vi "Timing.vi"(8 "error in":errorcluster, 9 "Stabilization Interval (s)":dbl, 10 "Time Left":refnum<notifier>, 11 "Message Queues out":T2) -> (0 "error out":errorcluster)   [LabVIEW 2014, in "Timing and Stabilization.lvlib"]
uses:
  Timing and Stabilization.lvlib
  MeasurementControl Message Queue Folder/All Message Queues.ctl
  MeasurementControl Message Queue Folder/Message Cluster.ctl
  Time Left.ctl
  MeasurementControl Message Queue Folder/Enqueue Message (Single).vi
  MeasurementControl Message Queue Folder/MeasurementControl Message Queue.lvlib
panel:
  out "Cluster":T1
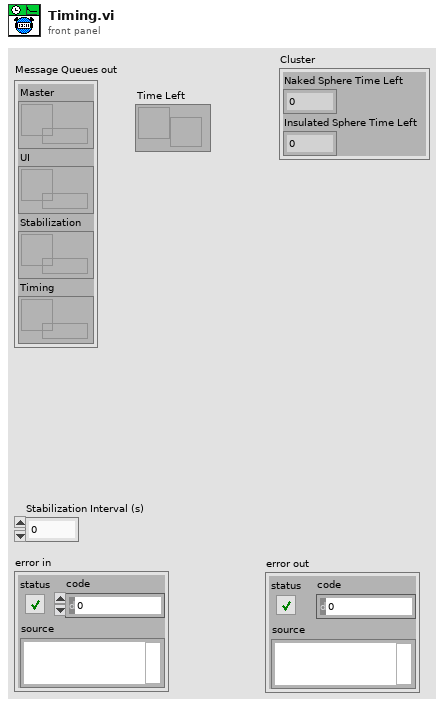
[diagram p1: front panel]
types:
  T1 = typedef "Time Left.ctl" = cluster{"Naked Sphere Time Left":dbl, "Insulated Sphere Time Left":dbl}
  T2 = typedef "MeasurementControl Message Queue.lvlib/All Message Queues.ctl" = cluster{"Master":refnum<queue>, "UI":refnum<queue>, "Stabilization":refnum<queue>, "Timing":refnum<queue>}
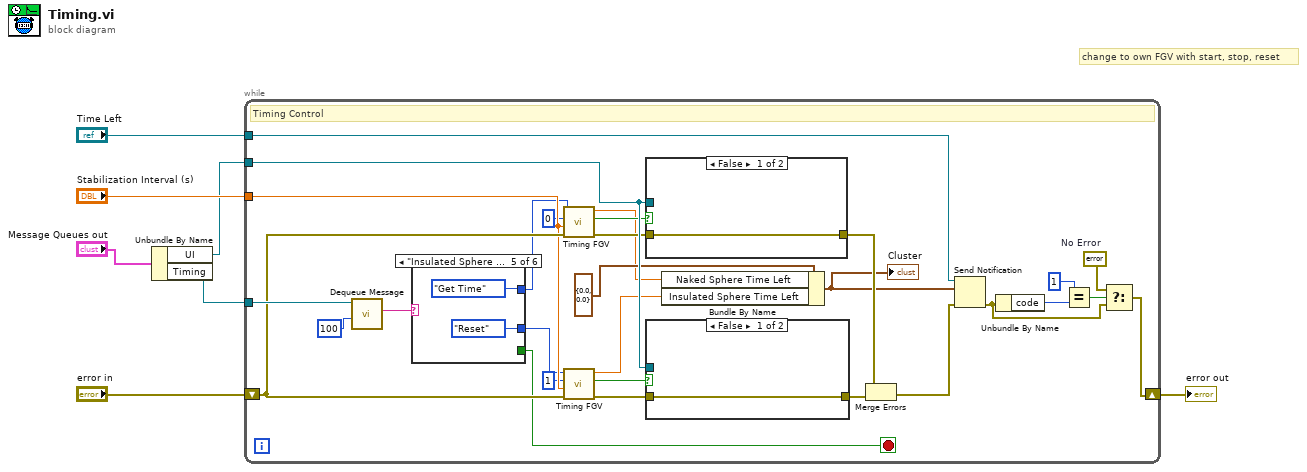
[diagram p0: block diagram]
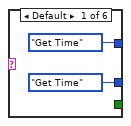
[diagram p2: hidden frame]
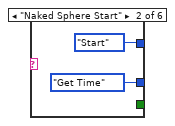
[diagram p3: hidden frame]
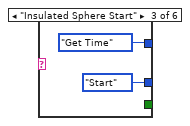
[diagram p4: hidden frame]
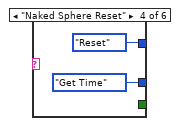
[diagram p5: hidden frame]
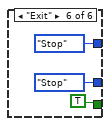
[diagram p6: hidden frame]
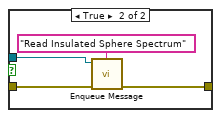
[diagram p7: hidden frame]
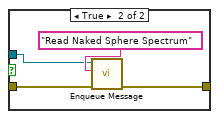
[diagram p8: hidden frame]
diagram:
  # "change to own FGV with start, stop, reset"
  n1 = Unbundle By Name("Message Queues out") -> ("UI"=w3:refnum<queue>, "Timing"=w2:refnum<queue>)
  n2 = while {
    shift-right: [w8] -> w5
    shift-left: "error in" -> [w31]
    tunnel: w2 -> [w36]
    tunnel: "Stabilization Interval (s)" -> [w28]
    tunnel: w3 -> [w33]
    tunnel: "Time Left" -> [w15]
    stop <- w20 stop-if-true
    w10 = errorcluster {"status"=FALSE, "code"=0, "source"=""}  # No Error
    # "Timing Control"
    n3 = call "Dequeue Message.vi"("timeout in ms (-1)"=100, "Message Queue"=w36) -> ("Message"=w23:string)  [unwired: 6 in, 3 out]
    n4 = case shown="\"Insulated Sphere Reset\"" w23 {
      tunnel: [enum16{"Start", "Stop", "Reset", "Get Time"}."Get Time" ("Method (Get Time)") enum16{"Start", "Stop", "Reset", "Get Time"}."Start" ("Method (Get Time)") enum16{"Start", "Stop", "Reset", "Get Time"}."Get Time" ("Method (Get Time)") enum16{"Start", "Stop", "Reset", "Get Time"}."Reset" ("Method (Get Time)") enum16{"Start", "Stop", "Reset", "Get Time"}."Get Time" ("Method (Get Time)") enum16{"Start", "Stop", "Reset", "Get Time"}."Stop" ("Method (Get Time)")] -> w22
      tunnel: [enum16{"Start", "Stop", "Reset", "Get Time"}."Get Time" ("Method (Get Time)") enum16{"Start", "Stop", "Reset", "Get Time"}."Get Time" ("Method (Get Time)") enum16{"Start", "Stop", "Reset", "Get Time"}."Start" ("Method (Get Time)") enum16{"Start", "Stop", "Reset", "Get Time"}."Get Time" ("Method (Get Time)") enum16{"Start", "Stop", "Reset", "Get Time"}."Reset" ("Method (Get Time)") enum16{"Start", "Stop", "Reset", "Get Time"}."Stop" ("Method (Get Time)")] -> w21
      tunnel: [_ _ _ _ _ TRUE] -> w20
      frame Default {
      }
      frame "Naked Sphere Start" {
      }
      frame "Insulated Sphere Start" {
      }
      frame "Naked Sphere Reset" {
      }
      frame "Insulated Sphere Reset" {
      }
      frame "Exit" {
      }
    }
    n5 = call "Timing FGV.vi"("error in (no error)"=w31, "Target time (s)"=w28, "Index"=0, "Method (Get Time)"=w22) -> ("error out"=w25:errorcluster, "Done"=w30:bool, "Time Remaining(s)"=w18:dbl)  [unwired: 5 in]
    n6 = call "Timing FGV.vi"("error in (no error)"=w31, "Target time (s)"=w28, "Index"=1, "Method (Get Time)"=w21) -> ("error out"=w24:errorcluster, "Done"=w29:bool, "Time Remaining(s)"=w17:dbl)  [unwired: 5 in]
    n7 = case shown="False" w30 {
      tunnel: [w55 w59] -> w35
      tunnel: w33 -> [_ w57]
      tunnel: w25 -> [w55 w56]
      frame False {
      }
      frame True {
        n8 = call-poly "Enqueue Message.vi"("error in (no error)"=w56, "Message"="Read Naked Sphere Spectrum", "Message Queue"=w57) -> ("error out"=w59:errorcluster)  [unwired: 7 in, 1 out]
      }
    }
    n9 = case shown="False" w29 {
      tunnel: [w50 w54] -> w34
      tunnel: w33 -> [_ w52]
      tunnel: w24 -> [w50 w51]
      frame False {
      }
      frame True {
        n10 = call-poly "Enqueue Message.vi"("error in (no error)"=w51, "Message"="Read Insulated Sphere Spectrum", "Message Queue"=w52) -> ("error out"=w54:errorcluster)  [unwired: 7 in, 1 out]
      }
    }
    n11 = Bundle By Name(cluster=T1 {"Naked Sphere Time Left"=0.0, "Insulated Sphere Time Left"=0.0} ("Cluster 2"), "Naked Sphere Time Left"=w18, "Insulated Sphere Time Left"=w17) -> (w16:T1)
    "Cluster" <- w16
    n12 = Merge Errors(w35, w34) -> (w14:errorcluster)
    n13 = Send Notification(notification=w16, notifier=w15, error in (no error)=w14) -> (error out=w9:errorcluster)  [unwired: 1 out]
    n14 = Unbundle By Name(w9) -> ("code"=w13:i32)
    n15 = Equal?(x=1, y=w13) -> (x = y?=w11:bool)
    n16 = Select(t=w10, s=w11, f=w9) -> (s? t:f=w8:errorcluster)
  }
  "error out" <- w5
